vi "testQuerySystemDefinitionFile.vi"(8 "error in (no error)":errorcluster, 11 "TestCase in":refnum<class "VeriStandTestUtilitiesTests.lvclass">) -> (0 "error out":errorcluster, 3 "TestCase out":refnum<class "VeriStandTestUtilitiesTests.lvclass">)   [LabVIEW 2027, in "VeriStandTestUtilitiesTests.lvclass"]
uses:
  VeriStandTestUtilitiesTests.lvclass
  Source/VeriStandTestUtilities/TargetInformation.ctl
  Source/VeriStandTestUtilities/ChassisInformation.ctl
  <vilib>/addons/_JKI Toolkits/VI Tester/TestCase.llb/TestCase.lvclass
  Source/VeriStandTestUtilities/VeriStandTestUtilities.lvlib
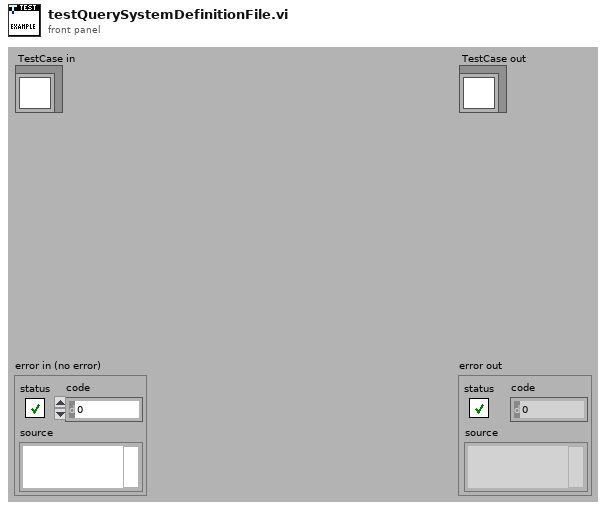
[diagram p1: front panel]
types:
  T1 = typedef "VeriStandTestUtilities.lvlib/TargetInformation.ctl" = cluster{"Name":string, "IP Address":string, "Operating System":string, "Target Rate":dbl, "Chassis List":T2[], "Custom Device List":string[]}
  T2 = typedef "VeriStandTestUtilities.lvlib/ChassisInformation.ctl" = cluster{"Name":string, "Devices":string[]}
  T3 = typedef "VeriStandTestUtilities.lvlib/SystemDefinitionInformation.ctl" = cluster{"Path":path, "Target Information List":T1[]}
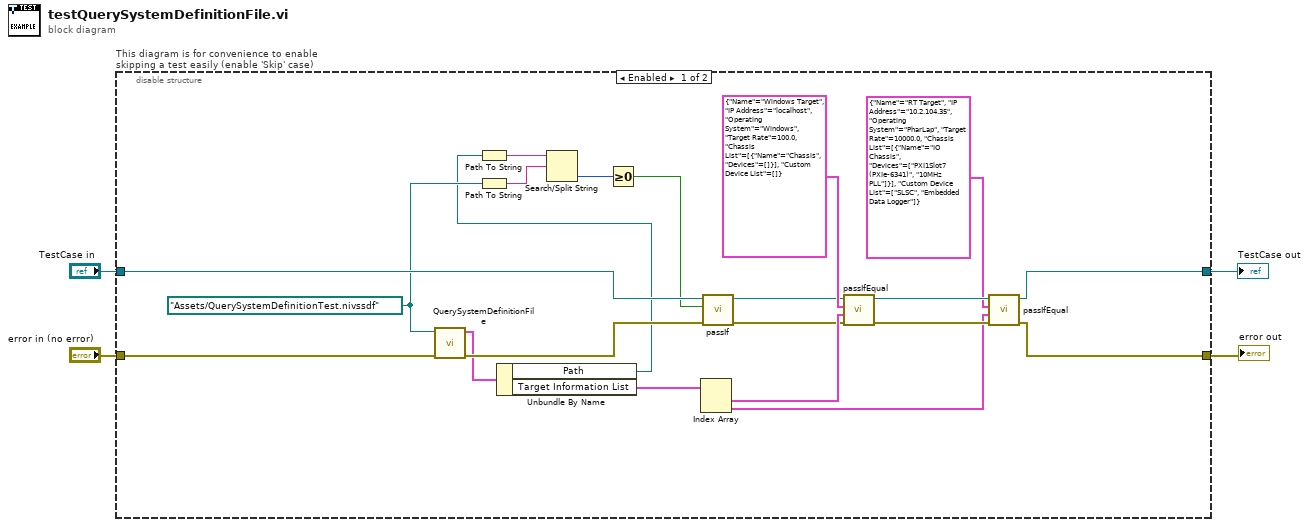
[diagram p0: block diagram]
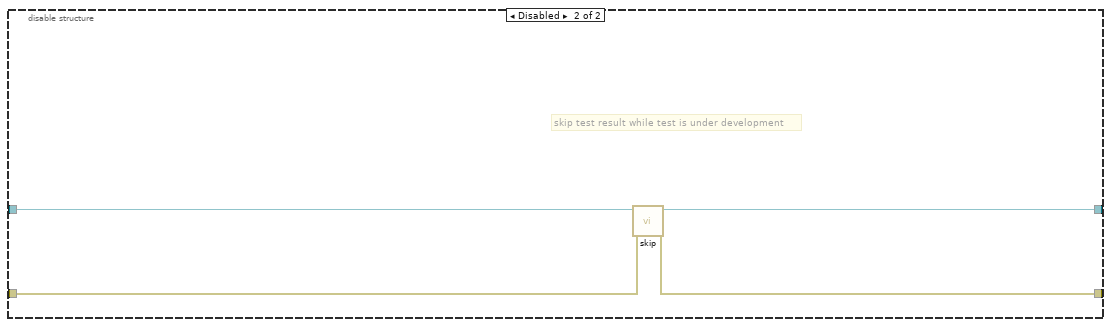
[diagram p2: hidden frame]
diagram:
  n1 = disable-structure "This diagram is for convenience to enable skipping a test easily (enable 'Skip' case)" shown="Enabled" {
    disable-tunnel: "TestCase in" -> [w12 w29]
    disable-tunnel: [w16 w27] -> w1
    disable-tunnel: [w19 w28] -> w3
    disable-tunnel: "error in (no error)" -> [w25 w26]
    frame Enabled {
      w10 = path "Assets/QuerySystemDefinitionTest.nivssdf" ("custom device xml path")
      n2 = call "QuerySystemDefinitionFile.vi"("error in (no error)"=w25, "System Definiton File in"=w10) -> ("error out"=w22:errorcluster, "System Definition Information out"=w15:T3)  [unwired: 8 in]
      n3 = Path To String(path=w10) -> (string=w7:string)
      n4 = Unbundle By Name(w15) -> ("Path"=w9:path, "Target Information List"=w14:T1[])
      n5 = Path To String(path=w9) -> (string=w8:string)
      n6 = Search/Split String(string=w8, search string/char (-)=w7) -> (offset of match=w6:i32)  [unwired: 1 in, 2 out]
      n7 = Greater Or Equal To 0?(x=w6) -> (x >= 0?=w5:bool)
      n8 = Index Array(array=w14) -> (element #1=w23:T1, element #2=w17:T1)  [unwired: 2 in]
      n9 = call-dynamic "passIf.vi"("error in (no error)"=w22, "pass"=w5, "TestCase in"=w12) -> ("error out"=w13:errorcluster, "TestCase out"=w11:refnum<class "VeriStandTestUtilitiesTests.lvclass">)  [unwired: 7 in]
      n10 = call-dynamic "passIfEqual.vi"("error in (no error)"=w13, "y"=w23, "x"=T1 {"Name"="Windows Target", "IP Address"="localhost", "Operating System"="Windows", "Target Rate"=100.0, "Chassis List"=[{"Name"="Chassis", "Devices"=[]}], "Custom Device List"=[]} ("element"), "TestCase in"=w11) -> ("error out"=w20:errorcluster, "TestCase out"=w21:refnum<class "VeriStandTestUtilitiesTests.lvclass">)  [unwired: 6 in]
      n11 = call-dynamic "passIfEqual.vi"("error in (no error)"=w20, "y"=w17, "x"=T1 {"Name"="RT Target", "IP Address"="10.2.104.35", "Operating System"="PharLap", "Target Rate"=10000.0, "Chassis List"=[{"Name"="IO Chassis", "Devices"=["PXI1Slot7 (PXIe-6341)", "10MHz PLL"]}], "Custom Device List"=["SLSC", "Embedded Data Logger"]} ("element 2"), "TestCase in"=w21) -> ("error out"=w19:errorcluster, "TestCase out"=w16:refnum<class "VeriStandTestUtilitiesTests.lvclass">)  [unwired: 6 in]
    }
    frame Disabled {
      # "skip test result while test is under development"
      n12 = call <vilib>:"skip.vi"("error in (no error)"=w26, "TestCase in"=w29) -> ("error out"=w28:errorcluster, "TestCase out"=w27:refnum<class "VeriStandTestUtilitiesTests.lvclass">)  [unwired: 8 in]
    }
  }
  "error out" <- w3
  "TestCase out" <- w1
